vi "script_match_command.vi"(1 "Match":string, 2 "Valid commands":string[](array[string])) -> (0 "Command":string)   [LabVIEW 2010]
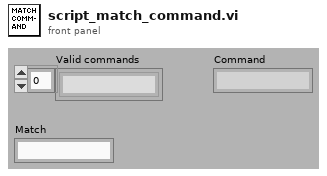
[diagram p1: front panel]
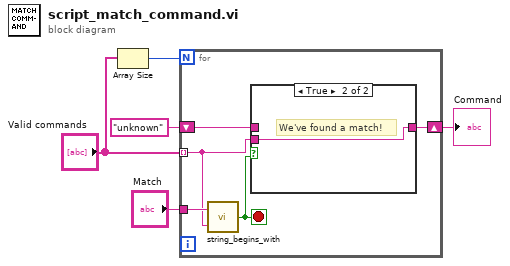
[diagram p0: block diagram]
diagram:
  n1 = Array Size(array="Valid commands") -> (size(s)=w1:i32)
  n2 = for {
    N: w1 -> [_]
    tunnel: "Valid commands" -> [w8] mode=indexing
    shift-right: [w7] -> w5
    shift-left: "unknown" -> [w6]
    tunnel: "Match" -> [w10]
    stop <- w9 stop-if-true
    n3 = call "string_begins_with.vi"("String to compare"=w8, "Beginning string"=w10) -> ("Begins with?"=w9:bool)
    n4 = case shown="True" w9 {
      tunnel: w8 -> [_ w12]
      tunnel: [w11 w12] -> w7
      tunnel: w6 -> [w11 _]
      frame False {
      }
      frame True {
        # "We've found a match!"
      }
    }
  }
  "Command" <- w5
